vi "InsertPatientIDIntoList.vi"(8 "error in (no error)":errorcluster, 10 "CPR Number":string, 11 "ListBox in":refnum<vi>) -> (0 "error out":errorcluster, 2 "CPR Number Out":string, 3 "ListBox out":refnum<vi>)   [LabVIEW 2013, in "main.lvlib"]
uses:
  main.lvlib
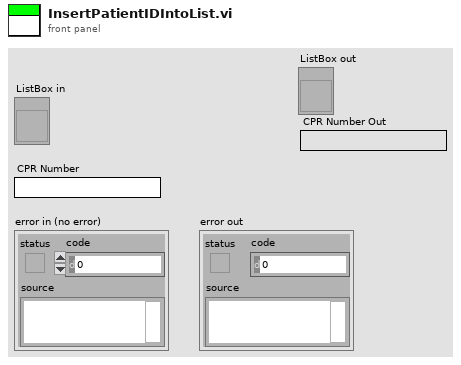
[diagram p1: front panel]
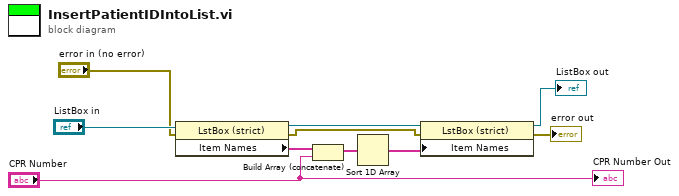
[diagram p0: block diagram]
diagram:
  n1 = property class="LstBox (strict)"(reference="ListBox in", error in="error in (no error)") -> (reference out=w5:refnum<vi>, error out=w7:errorcluster, "Item Names"=w2:string[])
  n2 = Build Array (concatenate)(w2, "CPR Number") -> (w4:string[])
  n3 = Sort 1D Array(array=w4) -> (sorted array=w6:string[])
  n4 = property class="LstBox (strict)"(reference=w5, error in=w7, "Item Names"=w6) -> (reference out=→"ListBox out":refnum<vi>, error out=→"error out":errorcluster)
  "CPR Number Out" <- "CPR Number"
